vi "Get New Control Position.vi"(8 "panel bounds":T1, 9 "边界":T3, 10 "位置":T2) -> (2 "位置":T2 caption="new position")   [LabVIEW 2024, in "Naughty Button.xctl"]
doc: "本VI是为《我和LabVIEW》一书编写的示例。\n关于本书的介绍请参考网页：\nhttp://ruanqizhen.spaces.live.com/blog/cns!5852D4F797C53FB6!4310.entry"
uses:
  Naughty Button.xctl
  <vilib>/Utility/miscctls.llb/LVPositionTypeDef.ctl
  <vilib>/Utility/miscctls.llb/LVBoundsTypeDef.ctl
  <vilib>/Utility/miscctls.llb/LVRectTypeDef.ctl
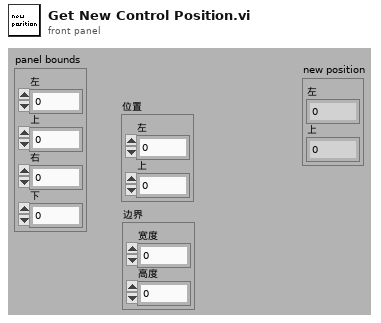
[diagram p1: front panel]
types:
  T1 = typedef "LVRectTypeDef.ctl" = cluster{"Left":i16, "Top":i16, "Right":i16, "Bottom":i16}
  T2 = typedef "LVPositionTypeDef.ctl" = cluster{"Left":i32, "Top":i32}
  T3 = typedef "LVBoundsTypeDef.ctl" = cluster{"Width":u32, "Height":u32}
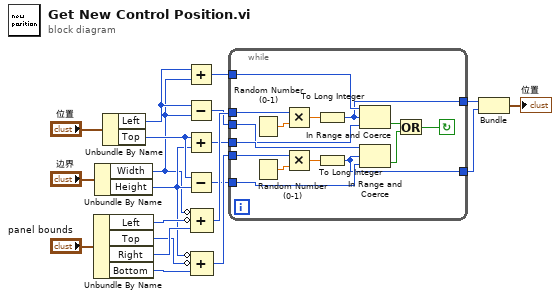
[diagram p0: block diagram]
diagram:
  n1 = Unbundle By Name("panel bounds") -> ("Left"=w12:i16, "Top"=w17:i16, "Right"=w18:i16, "Bottom"=w16:i16)
  n2 = Unbundle By Name("边界") -> ("Width"=w2:u32, "Height"=w5:u32)
  n3 = Unbundle By Name("位置") -> ("Left"=w3:i32, "Top"=w6:i32)
  n4 = Add(x=w3, y=w2) -> (x+y=w13:u32)
  n5 = Subtract(x=w3, y=w2) -> (x-y=w1:u32)
  n6 = Add(x=w6, y=w5) -> (x+y=w11:u32)
  n7 = Subtract(x=w6, y=w5) -> (x-y=w4:u32)
  n8 = Compound Arithmetic op=ADD(invert w2, invert w12, w18) -> (w15:u32)
  n9 = Compound Arithmetic op=ADD(invert w5, invert w17, w16) -> (w14:u32)
  n10 = while {
    tunnel: w15 -> [w35]
    tunnel: w14 -> [w33]
    tunnel: w13 -> [w30]
    tunnel: w11 -> [w28]
    tunnel: w4 -> [w27]
    tunnel: [w23] -> w10
    tunnel: [w22] -> w9
    tunnel: w1 -> [w21]
    stop <- w24 continue-if-true
    n11 = Random Number (0-1)() -> (number: 0 to 1=w34:dbl)
    n12 = Random Number (0-1)() -> (number: 0 to 1=w32:dbl)
    n13 = Multiply(x=w35, y=w34) -> (x*y=w31:dbl)
    n14 = Multiply(x=w33, y=w32) -> (x*y=w29:dbl)
    n15 = To Long Integer(number=w31) -> (32bit integer=w23:i32)
    n16 = To Long Integer(number=w29) -> (32bit integer=w22:i32)
    n17 = In Range and Coerce(upper limit=w30, x=w23, lower limit=w21) -> (In Range?=w25:bool)  [unwired: 1 out]
    n18 = In Range and Coerce(upper limit=w28, x=w22, lower limit=w27) -> (In Range?=w26:bool)  [unwired: 1 out]
    n19 = Or(x=w25, y=w26) -> (x .or. y?=w24:bool)
  }
  n20 = Bundle(w10, w9) -> (→"位置":cluster{i32, i32})  [unwired: 1 out]
